vi "Load and Sort Alarm tags from PSP.vi"(11 "Refnum in":refnum<k21>) -> (2 "Array 2":refnum<k21>[](array[refnum]), 3 "Array":T1[](array[typedef]))   [LabVIEW 2019]
uses:
  <vilib>/NI/Current Value Table/Type Defs/Single Tag.ctl
  <vilib>/NI/Current Value Table/Type Defs/Data Types.ctl
  <vilib>/NI/Current Value Table/Current Value Table.lvlib
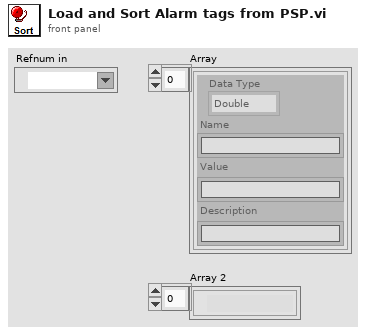
[diagram p1: front panel]
types:
  T1 = typedef "Current Value Table.lvlib/Single Tag.ctl" = cluster{"Data Type":T2, "Name":string, "Value":string, "Description":string}
  T2 = typedef "Current Value Table.lvlib/Data Types.ctl" = enum16{"Double", "Single", "I64", "I32", "I16", "I8", "U64", "U32", "U16", "U8", "String", "Boolean", "Array of U8", "Array of U16", "Array of U32", "Array of U64", "Array of I64", "Array of I32", "Array of I16", "Array of I8", "Array of Double", "Array of Single", "Array of Boolean", "Array of String"}
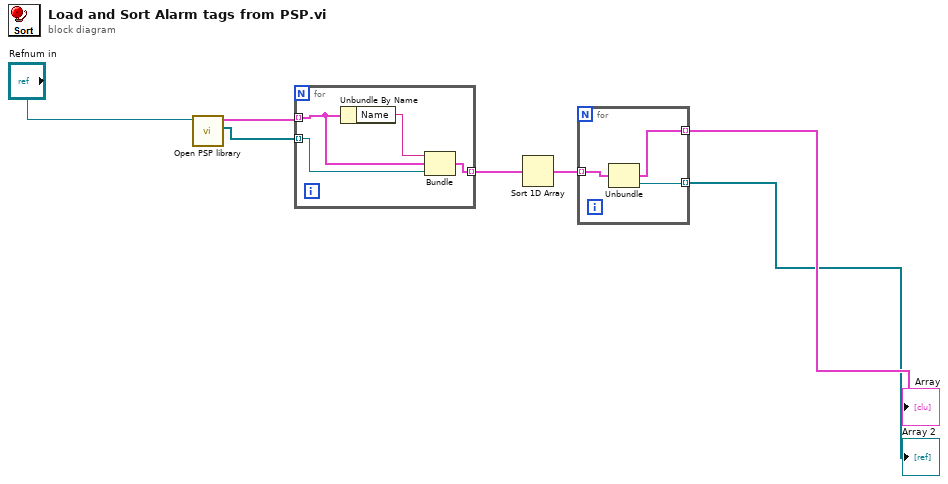
[diagram p0: block diagram]
diagram:
  n1 = call "Open PSP library.vi"("Refnum in"="Refnum in") -> ("Variables"=w3:refnum<k21>[], "CVT Array"=w2:T1[])  [unwired: 8 in, 1 out]
  n2 = for {
    tunnel: w2 -> [w10] mode=indexing
    tunnel: w3 -> [w9] mode=indexing
    tunnel: [w8] -> w4 mode=indexing
    n3 = Unbundle By Name(w10) -> ("Name"=w11:string)
    n4 = Bundle("Name"=w11, "Tag"=w10, w9) -> (w8:cluster{"Name":string, "Tag":T1, refnum<k21>})  [unwired: 1 in]
  }
  n5 = Sort 1D Array(array=w4) -> (sorted array=w5:cluster{"Name":string, "Tag":T1, refnum<k21>}[])
  n6 = for {
    tunnel: w5 -> [w14] mode=indexing
    tunnel: [w12] -> w7 mode=indexing
    tunnel: [w13] -> w6 mode=indexing
    n7 = Unbundle(w14) -> ("Tag"=w12:T1, w13:refnum<k21>)  [unwired: 1 out]
  }
  "Array" <- w7
  "Array 2" <- w6
